vi "TestGetLanguages.vi"(8 "error in (no error)":errorcluster) -> (0 "error out":errorcluster)   [LabVIEW 2017]
uses:
  src/API/JKI Simple Localization.lvlib
  <vilib>/addons/_JKI Toolkits/Caraya/classes/Test/Test.lvclass
  <vilib>/addons/_JKI Toolkits/Caraya/classes/Assert/Assert.lvclass
panel:
  # "See block diagram for unit tests of GetLanguages.vi"
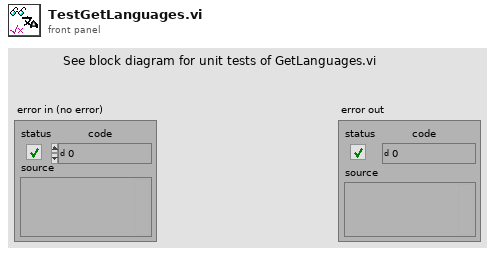
[diagram p1: front panel]
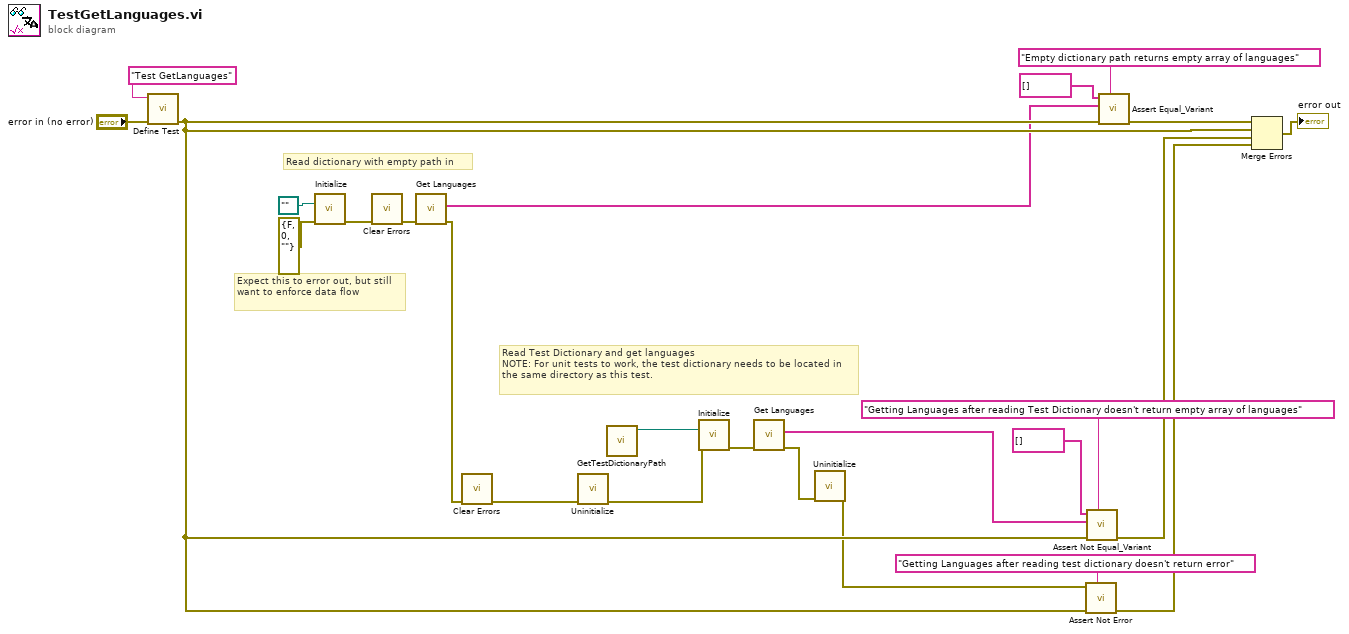
[diagram p0: block diagram]
diagram:
  # "Expect this to error out, but still want to enforce data flow"
  # "Read dictionary with empty path in"
  # "Read Test Dictionary and get languages \nNOTE: For unit tests to work, the test dictionary needs to be located in the same directory as this test."
  n1 = call <vilib>:"Define Test.vi"("error in (no error)"="error in (no error)", "Label (VI Title)"="Test GetLanguages") -> ("error out"=w18:errorcluster)  [unwired: 9 in]
  n2 = call "Initialize.vi"("Dictionary File Path"=path "", "error in"=errorcluster {"status"=FALSE, "code"=0, "source"=""}) -> ("error out"=w10:errorcluster)  [unwired: 10 in, 3 out]
  n3 = call <vilib>:"Clear Errors.vi"("error in (no error)"=w10) -> ("error out"=w11:errorcluster)  [unwired: 5 in, 1 out]
  n4 = call "Get Languages.vi"("error in"=w11) -> ("error out"=w6:errorcluster, "Languages"=w9:string[])  [unwired: 9 in]
  n5 = call <vilib>:"Clear Errors.vi"("error in (no error)"=w6) -> ("error out"=w5:errorcluster)  [unwired: 5 in, 1 out]
  n6 = call "Uninitialize.vi"("error in"=w5) -> ("error out"=w3:errorcluster)  [unwired: 10 in]
  n7 = call "GetTestDictionaryPath.vi"() -> ("Test Dictionary Path"=w4:path)  [unwired: 11 in]
  n8 = call "Initialize.vi"("Dictionary File Path"=w4, "error in"=w3) -> ("error out"=w8:errorcluster)  [unwired: 10 in, 3 out]
  n9 = call "Get Languages.vi"("error in"=w8) -> ("error out"=w2:errorcluster, "Languages"=w7:string[])  [unwired: 9 in]
  n10 = call "Uninitialize.vi"("error in"=w2) -> ("error out"=w1:errorcluster)  [unwired: 10 in]
  n11 = call <vilib>:"Assert Not Error.vi"("Label"="Getting Languages after reading test dictionary doesn't return error", "error in (no error)"=w18, "Not Error?"=w1) -> ("error out"=w12:errorcluster)  [unwired: 8 in]
  n12 = call <vilib>:"Assert Not Equal_Variant.vi"("Label"="Getting Languages after reading Test Dictionary doesn't return empty array of languages", "error in (no error)"=w18, "Y"=w7, "X"=string[] []) -> ("error out"=w13:errorcluster)  [unwired: 7 in]
  n13 = call <vilib>:"Assert Equal_Variant.vi"("Label"="Empty dictionary path returns empty array of languages", "error in (no error)"=w18, "Y"=w9, "X"=string[] []) -> ("error out"=w16:errorcluster)  [unwired: 7 in]
  n14 = Merge Errors(w16, w18, w13, w12) -> (→"error out":errorcluster)
